vi "ConnectedStatus.vi"(8 "error in (no error)":errorcluster, 11 "NhRegenGridSim in":refnum<class "NHRGridSim.lvclass">) -> (0 "error out":errorcluster, 2 "Connected?":bool, 3 "NhRegenGridSim out":refnum<class "NHRGridSim.lvclass">)   [LabVIEW 2018, in "AcPwrPlugins.lvlib" / "NHRGridSim.lvclass"]
doc: "This VI checks if the instrument is connected and passes along that connected status."
uses:
  NHRGridSim.lvclass
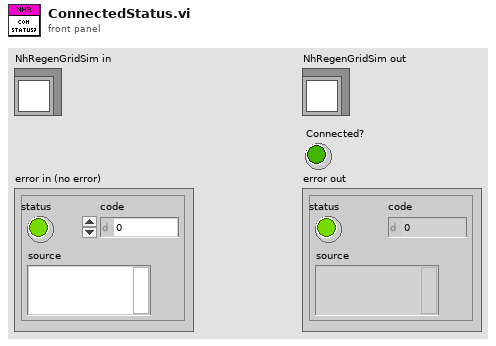
[diagram p1: front panel]
types:
  T1 = typedef "AcPwrPlugins.lvlib/NHRGridSim.lvclass/NHRGrid_Device(s)Settings.ctl" = cluster{"MeasName":string, "Hardware":T2}
  T2 = typedef "AcPwrPlugins.lvlib/NHRGridSim.lvclass/NHRGrid_Hardware.ctl" = cluster{"Handle":string, "Reset":bool, "Mode":T3, "ID Query":bool, "Logical Instrument":T4, "Connected":bool}
  T3 = typedef "AcPwrPlugins.lvlib/NHRGridSim.lvclass/NHRGrid_Modes.ctl" = u8
  T4 = typedef "AcPwrPlugins.lvlib/NHRGridSim.lvclass/NHRGrid_Logical_Instrument.ctl" = cluster{"Name":string, "Vout (V)":dbl, "I limit (A)":dbl, "P limit (W)":dbl, "FreqOut (Hz)":dbl, "Ranges":cluster{"Voltage (V)":u16, "Current (A)":u16}, "Configure Instrument":u16, "Aperture (cycles)":i32, "AC Wave Shape":u16, "VType":string, "IType":string, "Phases":T5, "Slew Rates":T6, "Safety Trips":T7}[]
  T5 = typedef "AcPwrPlugins.lvlib/NHRGridSim.lvclass/NHRGrid_Phases.ctl" = cluster{"A-Volts (V)":dbl, "B-Volts (V)":dbl, "C-Volts (V)":dbl, "A-Curr (A)":dbl, "B-Curr (A)":dbl, "C-Curr (A)":dbl, "A-Power (W)":dbl, "B-Power (W)":dbl, "C-Power (W)":dbl, "Change at (Deg)":dbl, "B-Angle (Deg)":dbl, "C-Angle (Deg)":dbl}
  T6 = typedef "AcPwrPlugins.lvlib/NHRGridSim.lvclass/NHRGrid_SlewRates.ctl" = cluster{"Vmax (V/s)":dbl, "Vmin (V/s)":dbl, "Imax (A/s)":dbl, "Imin (A/s)":dbl, "Pmax (W/s)":dbl, "Pmin (W/s)":dbl, "Freq Max (Hz/s)":dbl, "Freq Min (Hz/s)":dbl, "Phase Angle Max (Deg/s)":dbl, "Phase Angle Min (Deg/s)":dbl}
  T7 = typedef "AcPwrPlugins.lvlib/NHRGridSim.lvclass/NHRGrid_SafetyTrips.ctl" = cluster{"Vmax (V)":dbl, "Vmin (V)":dbl, "Vmax Time (s)":dbl, "Vmin Time (s)":dbl, "Imax Source (A)":dbl, "Imax Sink (A)":dbl, "Imax Source Time (s)":dbl, "Imax Sink Time (s)":dbl, "Pmax Source (W)":dbl, "Pmax Sink (W)":dbl, "Pmax Source Time (s)":dbl, "Pmax Sink Time (s)":dbl, "Absolute Volt Peak":dbl, "Enable Volt Peak":bool, "Absolute Curr Peak":dbl, "Enable Curr Peak":bool}
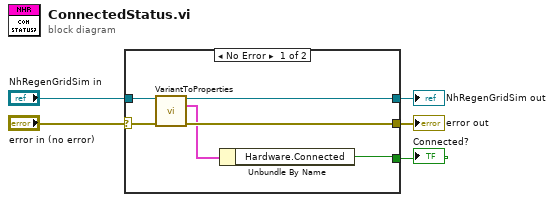
[diagram p0: block diagram]
diagram:
  n1 = case shown="No Error" "error in (no error)" {
    selector: "error in (no error)" -> [w10 w12]
    tunnel: "NhRegenGridSim in" -> [w11 w13]
    tunnel: [w8 w13] -> w3
    tunnel: [w9 w12] -> w2
    tunnel: [w6 _] -> w1
    frame No Error {
      n2 = call "VariantToProperties.vi"("NHRGridSim in"=w11, "error in (no error)"=w10) -> ("NHRGridSim out"=w8:refnum<class "NHRGridSim.lvclass">, "Device(s)Settings"=w7:T1, "error out"=w9:errorcluster)  [unwired: 8 in, 3 out]
      n3 = Unbundle By Name(w7) -> ("Hardware.Connected"=w6:bool)
    }
    frame Error {
    }
  }
  "error out" <- w2
  "NhRegenGridSim out" <- w3
  "Connected?" <- w1
